vi "Find RT Targets.vi"(8 "error in (no error)":errorcluster, 11 "Project Sync Tools in":refnum<class "Project Sync Tools.lvclass">) -> (0 "error out":errorcluster, 1 "RT Targets names":string[](array[string]), 2 "RT Targets refs":refnum<vi>[](array[refnum]), 3 "Project Sync Tools out":refnum<class "Project Sync Tools.lvclass">)   [LabVIEW 2019, in "Project Sync Tools.lvclass"]
uses:
  Project Sync Tools.lvclass
  Project Sync Tools.lvclass/Project Sync Tools.ctl
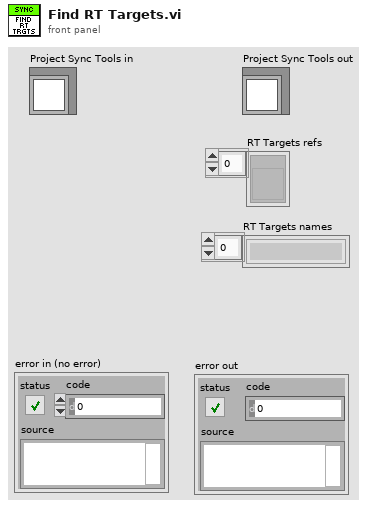
[diagram p1: front panel]
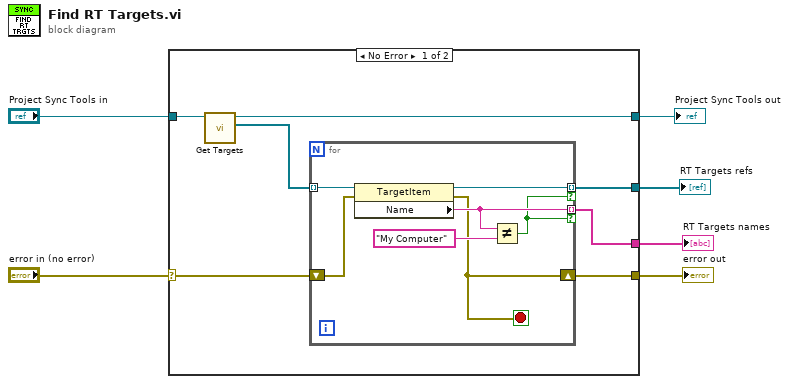
[diagram p0: block diagram]
diagram:
  n1 = case shown="No Error" "error in (no error)" {
    selector: "error in (no error)" -> [w8 w21]
    tunnel: [w13 w22] -> w6
    tunnel: "Project Sync Tools in" -> [w11 w22]
    tunnel: [w10 _] -> w4
    tunnel: [w9 _] -> w3
    tunnel: [w7 w21] -> w1
    frame No Error {
      n2 = call "Get Targets.vi"("Project Sync Tools in"=w11) -> ("Targets"=w12:refnum<vi>[], "Project Sync Tools out"=w13:refnum<class "Project Sync Tools.lvclass">)  [unwired: 9 in]
      n3 = for {
        tunnel: w12 -> [w20] mode=indexing
        tunnel: [w14] -> w10 mode=indexing if=w17
        tunnel: [w18] -> w9 mode=indexing if=w17
        shift-right: [w15] -> w7
        shift-left: w8 -> [w16]
        stop <- w15 stop-if-true
        n4 = property class="TargetItem"(reference=w20, error in=w16) -> (reference out=w14:refnum<vi>, error out=w15:errorcluster, "Name"=w18:string)
        n5 = Not Equal?(x=w18, y="My Computer") -> (x != y?=w17:bool)
      }
    }
    frame Error {
    }
  }
  "Project Sync Tools out" <- w6
  "RT Targets refs" <- w4
  "RT Targets names" <- w3
  "error out" <- w1
